vi "GetLatestExport.vi"(2 "error in":errorcluster, 3 "Export Root":path=path "\\\\limbo\\exports/labviewrt/Core/rt_exec/export") -> (0 "error out":errorcluster, 1 "Latest Root":path)   [LabVIEW 2011]
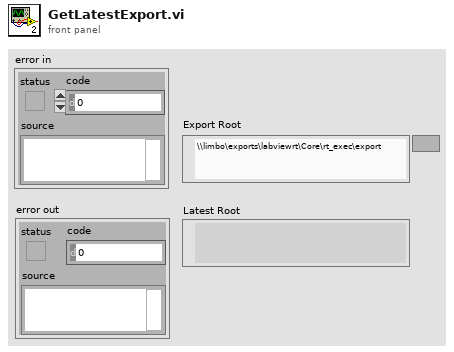
[diagram p1: front panel]
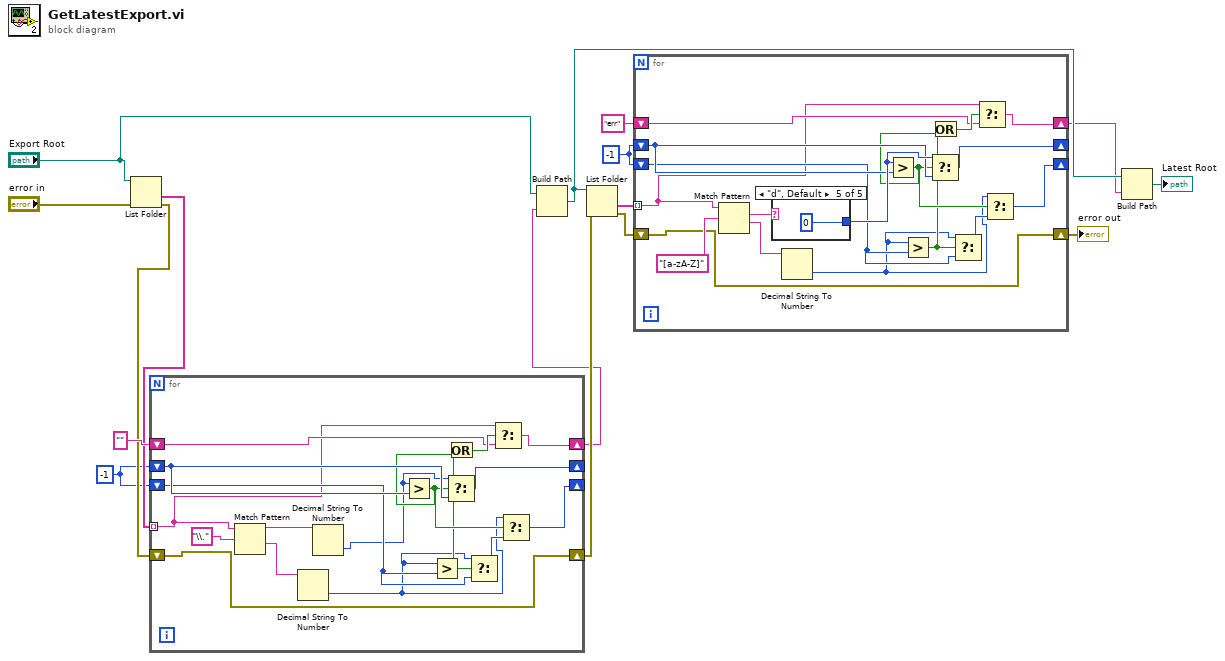
[diagram p0: block diagram]
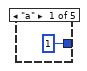
[diagram p2: hidden frame]
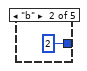
[diagram p3: hidden frame]
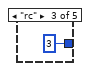
[diagram p4: hidden frame]
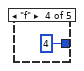
[diagram p5: hidden frame]
diagram:
  w1 = -1
  w11 = -1
  n1 = List Folder(path="Export Root", error in="error in") -> (folder names=w5:string[], error out=w4:errorcluster)  [unwired: 2 in, 2 out]
  n2 = for {
    tunnel: w5 -> [w23] mode=indexing
    shift-right: [w22] -> w3
    shift-left: w4 -> [w22]
    shift-right: [w24] -> w2
    shift-left: "" -> [w25]
    shift-right: [w30] -> _
    shift-left: w1 -> [w31]
    shift-right: [w18] -> _
    shift-left: w1 -> [w29]
    n3 = Match Pattern(string=w23, regular expression="\\.") -> (before substring=w21:string, after substring=w32:string)  [unwired: 1 in, 2 out]
    n4 = Decimal String To Number(string=w32) -> (number=w17:i32)  [unwired: 2 in, 1 out]
    n5 = Decimal String To Number(string=w21) -> (number=w20:i32)  [unwired: 2 in, 1 out]
    n6 = Greater?(x=w20, y=w31) -> (0:w28:bool)
    n7 = Greater?(x=w17, y=w29) -> (0:w27:bool)
    n8 = Select(t=w20, s=w28, f=w31) -> (s? t:f=w30:i32)
    n9 = Or(x=w27, y=w28) -> (x .or. y?=w26:bool)
    n10 = Select(t=w17, s=w27, f=w29) -> (s? t:f=w19:i32)
    n11 = Select(t=w23, s=w26, f=w25) -> (s? t:f=w24:string)
    n12 = Select(t=w17, s=w28, f=w19) -> (s? t:f=w18:i32)
  }
  n13 = Build Path(base path="Export Root", name or relative path=w2) -> (appended path=w10:path)
  n14 = List Folder(path=w10, error in=w3) -> (folder names=w14:string[], error out=w13:errorcluster)  [unwired: 2 in, 2 out]
  n15 = for {
    tunnel: w14 -> [w38] mode=indexing
    shift-right: [w37] -> w7
    shift-left: w13 -> [w37]
    shift-right: [w39] -> w9
    shift-left: "err" ("result string") -> [w40]
    shift-right: [w45] -> _
    shift-left: w11 -> [w46]
    shift-right: [w35] -> _
    shift-left: w11 -> [w44]
    n16 = Match Pattern(string=w38, regular expression="[a-zA-Z]") -> (match substring=w49:string, after substring=w48:string)  [unwired: 1 in, 2 out]
    n17 = case shown="\"d\", Default" w49 {
      tunnel: [1 2 3 4 0] -> w47
      frame "a" {
      }
      frame "b" {
      }
      frame "rc" {
      }
      frame "f" {
      }
      frame "d", Default {
      }
    }
    n18 = Decimal String To Number(string=w48) -> (number=w34:i32)  [unwired: 2 in, 1 out]
    n19 = Greater?(x=w47, y=w46) -> (0:w43:bool)
    n20 = Greater?(x=w34, y=w44) -> (0:w42:bool)
    n21 = Select(t=w47, s=w43, f=w46) -> (s? t:f=w45:i32)
    n22 = Or(x=w42, y=w43) -> (x .or. y?=w41:bool)
    n23 = Select(t=w34, s=w42, f=w44) -> (s? t:f=w36:i32)
    n24 = Select(t=w38, s=w41, f=w40) -> (s? t:f=w39:string)
    n25 = Select(t=w34, s=w43, f=w36) -> (s? t:f=w35:i32)
  }
  "error out" <- w7
  n26 = Build Path(base path=w10, name or relative path=w9) -> (appended path=→"Latest Root":path)
